vi "HV Load Test_production_SPIN2.vi"(5 "Published_Data_ID":string="HV39_", 7 "Reg0_State":string="State00", 10 "HV_Load_Steps_uA":dbl[](array[numeric])=[0.0, 5.0, 8.0, 10.0] format="%#_6p", 11 "Semiconductor Module Context":T1) -> (0 "error out":errorcluster)   [LabVIEW 2013]
uses:
  <vilib>/NI_TestStand_SemiconductorModule/NI_TestStand_Semiconductor_Module.lvlibp/PinMap/General/SemiconductorModuleContext.ctl
  <vilib>/NI_TestStand_SemiconductorModule/NI_TestStand_Semiconductor_Module.lvlibp/PinMap/DC Power/PinsToNIDCPowerSessions.vi
  <vilib>/NI_TestStand_SemiconductorModule/NI_TestStand_Semiconductor_Module.lvlibp/PinMap/Deprecated/PublishDataDoubleMultiplePinsSingleInstrument.vi
  <vilib>/NI_TestStand_SemiconductorModule/NI_TestStand_Semiconductor_Module.lvlibp
panel:
  out "current measurements":dbl[][](array[numeric]) format="%#_6p"
  out "voltage measurements":dbl[][](array[numeric])
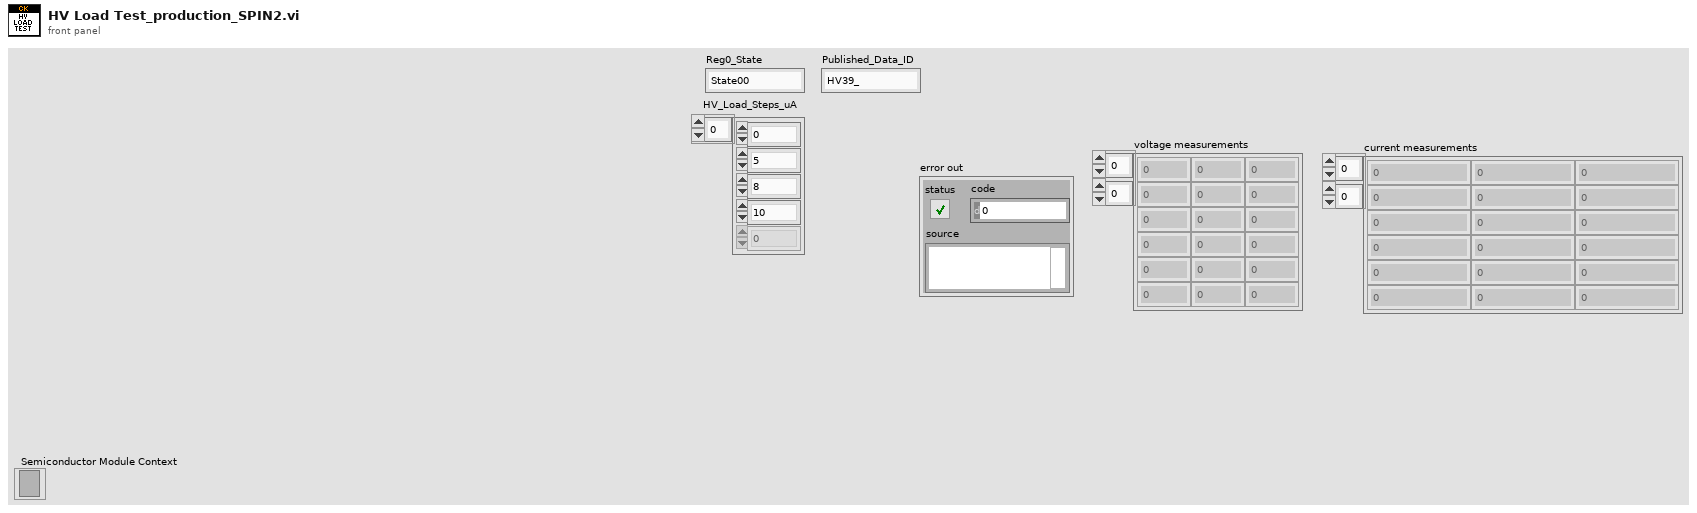
[diagram p1: front panel]
types:
  T1 = typedef "NI_TestStand_Semiconductor_Module.lvlibp/SemiconductorModuleContext.ctl" = refnum<k7>
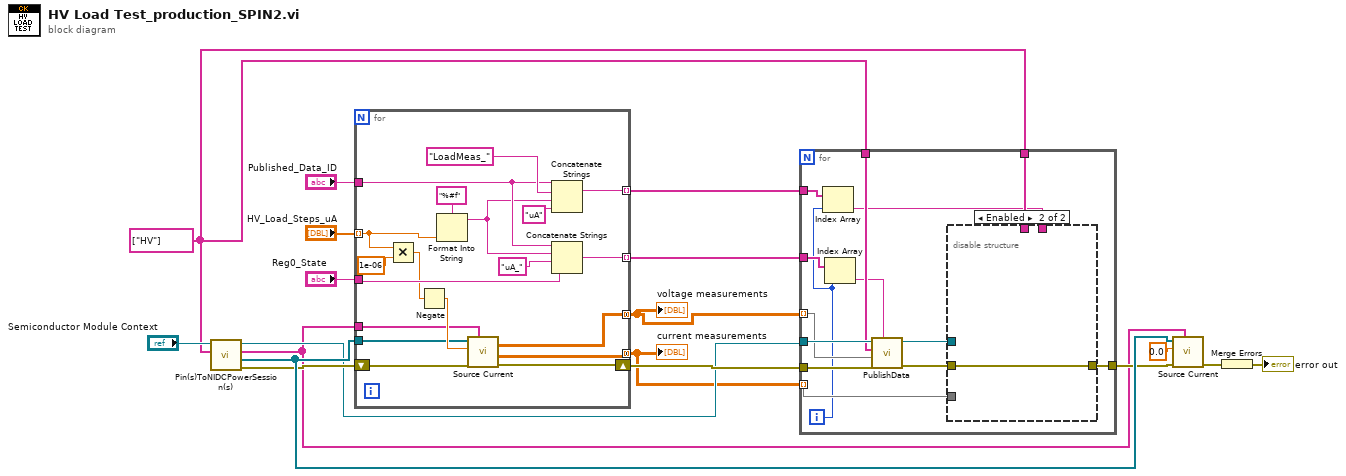
[diagram p0: block diagram]
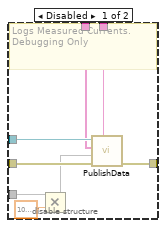
[diagram p2: hidden frame]
diagram:
  w6 = string[] ["HV"] ("Pins")
  n1 = call-poly <vilib>:"Pin(s)ToNIDCPowerSession(s).vi"("Pins"=w6, "Semiconductor Module Context"="Semiconductor Module Context") -> ("error out"=w14:errorcluster, "Instrument Sessions"=w16:refnum<k15>[], "Channel Lists"=w8:string[], "Semiconductor Module Context Out"=w9:T1)  [unwired: 5 in, 1 out]
  n2 = for {
    tunnel: w8 -> [w26]
    tunnel: "HV_Load_Steps_uA" -> [w20] mode=indexing
    tunnel: w16 -> [w23]
    shift-right: [w24] -> w11
    shift-left: w14 -> [w25]
    tunnel: "Published_Data_ID" -> [w30]
    tunnel: "Reg0_State" -> [w35]
    tunnel: [w34] -> w7 mode=concatenating
    tunnel: [w33] -> w2 mode=indexing
    tunnel: [w32] -> w5 mode=concatenating
    tunnel: [w29] -> w3 mode=indexing
    n3 = Multiply(x=w20, y=1e-06) -> (x*y=w22:dbl)
    n4 = Negate(x=w22) -> (-x=w36:dbl)
    n5 = Format Into String(format string="%#f", w20) -> (resulting string=w19:string)  [unwired: 2 in, 1 out]
    n6 = call "Source Current.vi"("Channel Lists"=w26, "error in (no error)"=w25, "current level"=w36, "Instrument Sessions In"=w23) -> ("error out"=w24:errorcluster, "current measurements"=w32:dbl[][], "voltage measurements"=w34:dbl[][])  [unwired: 4 in, 1 out]
    n7 = Concatenate Strings(w30, "LoadMeas_" ("string"), w19, "uA" ("string")) -> (w29:string)
    n8 = Concatenate Strings(w30, w19, "uA_" ("string"), w35) -> (w33:string)
  }
  "voltage measurements" <- w7
  "current measurements" <- w5
  n9 = for {
    tunnel: w11 -> [w51]
    tunnel: [w47] -> w10
    tunnel: w9 -> [w50]
    tunnel: w7 -> [w49] mode=indexing
    tunnel: w6 -> [w48]
    tunnel: w6 -> [w44]
    tunnel: w5 -> [w43] mode=indexing
    tunnel: w2 -> [w42]
    tunnel: w3 -> [w41]
    i -> [w38]
    n10 = Index Array(array=w41, index=w38) -> (element=w40:string)
    n11 = Index Array(array=w42, index=w38) -> (element=w39:string)
    n12 = call-poly <vilib>:"PublishData.vi"("Measurement Id"=w39, "error in (no error)"=w51, "Data In"=w49, "Pins"=w48, "Semiconductor Module Context"=w50) -> ("error out"=w46:errorcluster, "Semiconductor Module Context Out"=w45:T1)  [unwired: 5 in]
    n13 = disable-structure shown="Enabled" {
      disable-tunnel: [w59 w60] -> w47
      disable-tunnel: w46 -> [w58 w60]
      disable-tunnel: w45 -> [w57 _]
      disable-tunnel: w44 -> [w56 _]
      disable-tunnel: w43 -> [w53 _]
      disable-tunnel: w40 -> [w52 _]
      frame Disabled {
        # "Logs Measured Currents.\nDebugging Only"
        n14 = Multiply(x=w53, y=1000000.0) -> (x*y=w55:dbl[])
        n15 = call-poly <vilib>:"PublishData.vi"("Measurement Id"=w52, "error in (no error)"=w58, "Data In"=w55, "Pins"=w56, "Semiconductor Module Context"=w57) -> ("error out"=w59:errorcluster)  [unwired: 5 in, 1 out]
      }
      frame Enabled {
      }
    }
  }
  n16 = call "Source Current.vi"("Channel Lists"=w8, "error in (no error)"=w10, "current level"=0.0, "Instrument Sessions In"=w16) -> ("error out"=w1:errorcluster)  [unwired: 4 in, 3 out]
  n17 = Merge Errors(w1) -> (→"error out":errorcluster)
